vi "PH_gentec_Powermeter.ProcEvents.vi"(0 "i ref in":refnum<vi>, 5 "error in":errorcluster) -> (14 "i ref out":refnum<vi>, 19 "error out":errorcluster)   [LabVIEW 2014, in "PH_gentec_Powermeter.lvlib"]
doc: "This method is used to define the events the object will listen to. Add your own events here."
uses:
  PH_gentec_Powermeter.lvlib
  CSCore/BaseProcess/BaseProcess.event definition.ctl
  CSCore/CAEObj/CAEObj.event definition.ctl
  CSCore/BaseProcess/BaseProcess.descriptor string definition.ctl
  CSCore/BaseProcess/BaseProcess.lvlib
  CSCore/CAEObj/CAEObj.lvlib
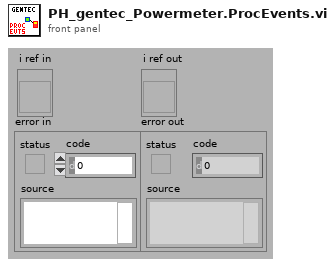
[diagram p1: front panel]
types:
  T1 = typedef "BaseProcess.lvlib/BaseProcess.event definition.ctl" = cluster{"CAEEvtDef":T2, "Data Descriptor":T3}
  T2 = typedef "CAEObj.lvlib/CAEObj.event definition.ctl" = cluster{"URL":string, "enable":bool, "ignoreResID":bool}
  T3 = typedef "BaseProcess.lvlib/BaseProcess.descriptor string definition.ctl" = string
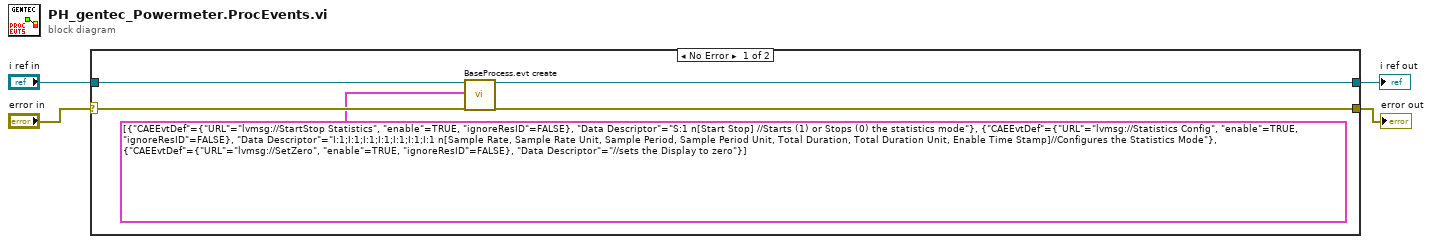
[diagram p0: block diagram]
diagram:
  n1 = case shown="No Error" "error in" {
    selector: "error in" -> [w7 w10]
    tunnel: "i ref in" -> [w6 w11]
    tunnel: [w9 w11] -> w3
    tunnel: [w8 w10] -> w2
    frame No Error {
      n2 = call "BaseProcess.evt create.vi"("i ref in"=w6, "newEvents"=T1[] [{"CAEEvtDef"={"URL"="lvmsg://StartStop Statistics", "enable"=TRUE, "ignoreResID"=FALSE}, "Data Descriptor"="S:1 n[Start Stop] //Starts (1) or Stops (0) the statistics mode"}, {"CAEEvtDef"={"URL"="lvmsg://Statistics Config", "enable"=TRUE, "ignoreResID"=FALSE}, "Data Descriptor"="I:1;I:1;I:1;I:1;I:1;I:1;I:1 n[Sample Rate, Sample Rate Unit, Sample Period, Sample Period Unit, Total Duration, Total Duration Unit, Enable Time Stamp]//Configures the Statistics Mode"}, {"CAEEvtDef"={"URL"="lvmsg://SetZero", "enable"=TRUE, "ignoreResID"=FALSE}, "Data Descriptor"="//sets the Display to zero"}] ("new events(V3.0)"), "error in (no error)"=w7) -> ("i ref out"=w9:refnum<vi>, "error out"=w8:errorcluster)  [unwired: 13 in, 2 out]
    }
    frame Error {
    }
  }
  "i ref out" <- w3
  "error out" <- w2
